vi "Configure Measurement Histogram (N Cycle Jitter).vi"(0 "VISA resource name":refnum<visa-resource-name>, 1 "Enable Measurement Histogram (Enable)":bool=TRUE, 2 "Number Cycle (5)":u32=5, 3 "Start Cycle (1)":u32=1, 5 "Channel (1: Channel 1)":i32(ring)=1 items=["Channel 1"=1, "Channel 2"=2, "Channel 3"=3, "Channel 4"=4, "Function 1"=5, "Function 2"=6, "Function 3"=7, "Function 4"=8, "Memory 1"=9, "Memory 2"=10, "Memory 3"=11, "Memory 4"=12], 7 "Edge (0: Rising)":i32(ring) items=["Rising", "Falling"], 11 "error in (no error)":errorcluster) -> (4 "VISA resource name out":refnum<visa-resource-name>, 15 "error out":errorcluster)   [LabVIEW 2012, in "Agilent 8000 Series.lvlib"]
doc: "Configures the N C Jitter measurement and enables the Measurement Histogram Jitter analysis on it.\n\n<B>Note:</B>\nCalling this VI disables all previously enabled measurements and clears existing measurement results from display."
uses:
  Agilent 8000 Series.lvlib
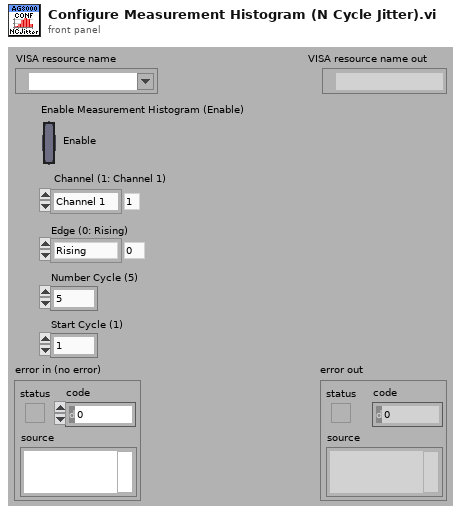
[diagram p1: front panel]
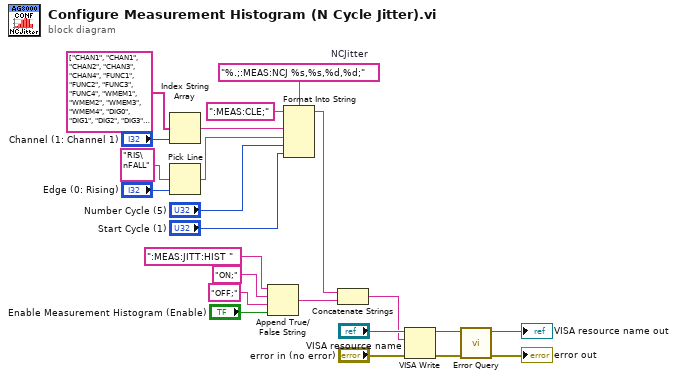
[diagram p0: block diagram]
diagram:
  w16 = "%.;:MEAS:NCJ %s,%s,%d,%d;"  # NCJitter
  n1 = Index String Array(1:"Channel (1: Channel 1)", 2:string[] ["CHAN1", "CHAN1", "CHAN2", "CHAN3", "CHAN4", "FUNC1", "FUNC2", "FUNC3", "FUNC4", "WMEM1", "WMEM2", "WMEM3", "WMEM4", "DIG0", "DIG1", "DIG2", "DIG3", "DIG4", "DIG5", "DIG6", "DIG7", "DIG8", "DIG9", "DIG10", "DIG11", "DIG12", "DIG13", "DIG14", "DIG15", "AUX", "LINE"]) -> (0:w14:string)  [unwired: 1 in]
  n2 = Pick Line(multi-line string="RIS\nFALL", line index="Edge (0: Rising)") -> (output string=w10:string)  [unwired: 1 in]
  n3 = Append True/False String(1:"Enable Measurement Histogram (Enable)", 2:"OFF;" ("false string"), 3:"ON;" ("true string"), 4:":MEAS:JITT:HIST " ("string (\"\")")) -> (0:w1:string)
  n4 = Format Into String(format string=w16, initial string=":MEAS:CLE;", w14, w10, "Number Cycle (5)", "Start Cycle (1)") -> (resulting string=w2:string)  [unwired: 1 in, 1 out]
  n5 = Concatenate Strings(w2, w1) -> (w3:string)
  n6 = VISA Write(VISA resource name="VISA resource name", write buffer=w3, error in (no error)="error in (no error)") -> (VISA resource name out=w19:refnum<visa-resource-name>, error out=w18:errorcluster)  [unwired: 1 out]
  n7 = call "Error Query.vi"("error in (no error)"=w18, "VISA resource name"=w19) -> ("error out"=→"error out":errorcluster, "VISA resource name out"=→"VISA resource name out":refnum<visa-resource-name>)  [unwired: 6 in, 2 out]
